vi "Realtime module.vi"() -> ()   [LabVIEW 2019]
uses:
  <vilib>/Platform/TimedLoop/XDataNode/timing_clust.ctl
  <vilib>/Platform/TimedLoop/XDataNode/nitl_modes.ctl
  <vilib>/Platform/TimedLoop/XDataNode/wakeup.ctl
  <vilib>/FPGAPlugInAG/myRIO-1900/niLvFpga_Open_myRIO-1900.vi
  <vilib>/rvi/interface/common/dynamic/niFpgaDynamicAddResources.vi
  <vilib>/Utility/error.llb/Error Cluster From Error Code.vi
  <vilib>/rvi/errors/niLvFpgaAdjustHostInterfaceError.vi
  <vilib>/FPGAPlugInAG/Dynamic/niLvFpga_Close_Dynamic.vi
  <vilib>/platform/TimedLoop/XDataNode/XDataNode.xnode
  <vilib>/rvi/interface/nirviOpenFPGA/nirviOpenFPGA.xnode
  FPGA Bitfiles/dcmotordynamomet_FPGATarget_FPGAmodule_FvbKT0KolIY.lvbitx
  FPGA module.vi
  <vilib>/rvi/interface/nirviMethod/nirviMethod.xnode
  <vilib>/rvi/interface/nirviCloseFPGA/nirviCloseFPGA.xnode
  <vilib>/FPGAPlugInAG/Dynamic/niLvFpga_ReadFifo_Dynamic.vi
  <vilib>/rvi/errors/niLvFpgaMergeErrorWithErrorCode.vi
  <vilib>/Platform/TimedLoop/XDataNode/XDNodeRunTimeDep.lvlib
  <vilib>/FPGAPlugInAG/Dynamic/niLvFpga_WriteFifo_Dynamic.vi
panel:
  in  "Ratio":sgl=0.4
  in  "Boolean":bool
  out "Error Chart":dynamicdata(graph)
  in  "Tab Control":T1(tab)
  out "?":dbl
  out "Slip":dbl(graph)
  out "?":dbl
  out "?":dbl
  out "AVG Speed (RPM)":dbl format="%#_5g"
  out "AVG Voltage Motor (V)":dbl format="%#_2g"
  out "AVG Voltage Battery (V)":dbl format="%#_4g"
  out "AVG Current Battery-Driver \nof Generator (A)":dbl format="%#_3g"
  out "AVG Current \nDriver-Generator (A)":dbl format="%#_2g"
  out "AVG Current Battery-Driver \nof Motor (A)":dbl format="%#_3g"
  out "AVG Current\nDriver-Motor (A)":dbl format="%#_3g"
  out "Lowpass Motor Voltage":dbl
  out "Current\nDriver-Generator (A)":dbl
  out "Current Battery-Driver\nof Generator (A)":dbl
  out "Current Battery-Driver\nof Motor (A)":dbl
  out "Current\nDriver-Motor (A)":dbl
  out "Generator Current Chart":dynamicdata(graph)
  in  "Generator\nCurrent (A)":dbl(slide) scale=0.0..40.0
  in  "Calibrated \nmax current":dbl=40.0
  in  "Motor\nVoltage (V)":dbl(slide) scale=0.0..24.0
  in  "Calibrated \nmax voltage":dbl=24.0
  out "Lowpass Battery Voltage":dbl
  out "Speed Chart":dynamicdata(graph)
  out "Voltage Chart":dynamicdata(graph)
  out "Motor Current Chart":dynamicdata(graph)
  out "AVG Motor Moment (Nm)":dbl format="%#_4g"
  out "AVG Generator Moment (Nm)":dbl format="%#_4g"
  out "Motor PID Chart":dynamicdata(graph)
  out "Generator PID Chart":dynamicdata(graph)
  out "b'":dbl
  out "a'":dbl
  out "b":dbl
  out "a":dbl
  in  "ELL":dbl=-0.8
  in  "EUL":dbl=0.8
  in  "EL1":dbl
  out "Error IN (G)":dbl
  out "Error OUT (G)":dbl
  out "Error In (M)":dbl
  out "Error OUT (M)":dbl
  in  "Alpha\nVoltage":dbl=0.05
  in  "Alpha\nCurrent":dbl=0.025
  in  "PID upper\n limit (G)":dbl
  in  "PID lower\n limit (G)":dbl=-1.0
  out "Output (G)":dbl
  out "PID (G)":dbl
  in  "I lower\nlimit (G)":dbl=-1.0
  in  "I upper\nlimit (G)":dbl
  out "D (G)":dbl
  out "I (G)":dbl
  out "P (G)":dbl
  in  "Kd (G)":dbl=0.001
  in  "Ki (G)":dbl=7.0
  in  "Kp (G)":dbl
  out "Output (M)":dbl
  in  "Kp (M)":dbl
  in  "Ki (M)":dbl=15.0
  in  "Kd (M)":dbl=0.01
  in  "I upper\nlimit (M)":dbl=1.0
  in  "I lower\nlimit (M)":dbl
  in  "PID lower\n limit (M)":dbl
  in  "PID upper\n limit (M)":dbl=1.0
  in  "PID Motor":bool=TRUE
  out "PID (M)":dbl
  in  "PID_Period\nMotor":dbl=0.005
  out "P (M)":dbl
  out "I (M)":dbl
  out "D (M)":dbl
  in  "PID Generator":bool=TRUE
  in  "PID_Period\nGenerator":dbl=0.005
  in  "Offset D-M":dbl
  in  "Offset B-D M":dbl
  in  "Offset D-G":dbl
  in  "Offset B-D G":dbl
  out "Output (Mot)":dbl
  out "C/Analog1":dbl
  out "C/Analog0":dbl
  out "A/Analog 3":dbl
  out "A/Analog2":dbl
  out "A/Analog1":dbl
  out "A/Analog0":dbl
  in  "C":dbl=5.1047
  in  "Min Channel C":dbl=-10.0
  in  "Min Channel A":dbl
  out "n samples":dbl
  out "Data 3":i32[](array[numeric]) caption="Data C/AI"
  in  "Max Channel C":dbl=10.0
  in  "B":dbl=-59.193
  in  "A":dbl=23.7
  in  "Max Channel A":dbl=5.0
  in  "Signal resolution":dbl=4095.0
  out "32bit integer generator":i32
  out "32bit integer motor":i32
  out "Samples":dbl
  out "Sum Bat Voltage":dbl
  out "Sum Mot Voltage":dbl
  out "Sum Bat-Dri of Gen":dbl
  out "Sum Bat-Dri of Mot":dbl
  out "Sum Generator":dbl
  out "Sum Motor":dbl
  out "Sum Speed":dbl
  in  "Encoder Resolution":dbl=16.0
  out "A/AI2":dbl
  out "A/AI3":dbl
  out "Executing Duration":u32
  out "Data":i32[](array[numeric])
  out "A/AI0":dbl
  out "A/AI1":dbl
  out "C/AI0":dbl
  out "Motor Voltage":dbl
  out "Bat-Dri Current (A) Mot":dbl
  out "Dri-Mot Current (A)":dbl
  out "Bat-Dri Current (A) Gen":dbl
  out "Dri-Gen Current (A)":dbl
  out "C/AI1":dbl
  out "Battery Voltage":dbl
  out "n speed":i32
  out "duration":i32
  out "Data Speed":i32[](array[numeric])
  out "Output (Gen)":dbl
  in  "Offset Motor Moment":dbl
  in  "Offset Generator Moment":dbl
  out "Motor Moment (Nm)":dbl format="%#_4g"
  out "Max Motor Moment":dbl
  out "Min Motor Moment":dbl
  out "Generator Moment (Nm)":dbl format="%#_4g"
  out "Max Gen Moment":dbl
  out "Min Gen Moment":dbl
  in  "alpha Motor moment":dbl=0.025
  in  "Lowpass Filter for Moment?":bool=TRUE
  in  "alpha Gen moment":dbl=0.025
  out "B/AI0":dbl
  out "B/AI1":dbl
  in  "Gain_Mot_Loadcell":dbl=3.6711
  in  "Offset_Mot_Loadcell":dbl=-8.6555
  in  "Gain_Gen_Loadcell":dbl=3.83101
  in  "Offset_Gen_Loadcell":dbl=-9.60463
  out "Sum ADC Mot Loadcell":dbl
  out "Sum ADC Gen Loadcell":dbl
  out "Sum Mot Moment":dbl
  out "Sum Gen Moment":dbl
  out "AVG ADC Mot Loadcell (V)":dbl
  out "AVG ADC Gen Loadcell (V)":dbl
  out "ADC B/AI0":dbl
  out "ADC B/AI1":dbl
  out "Motor Moment Chart":dbl(graph)
  out "Generator Moment Chart":dbl(graph)
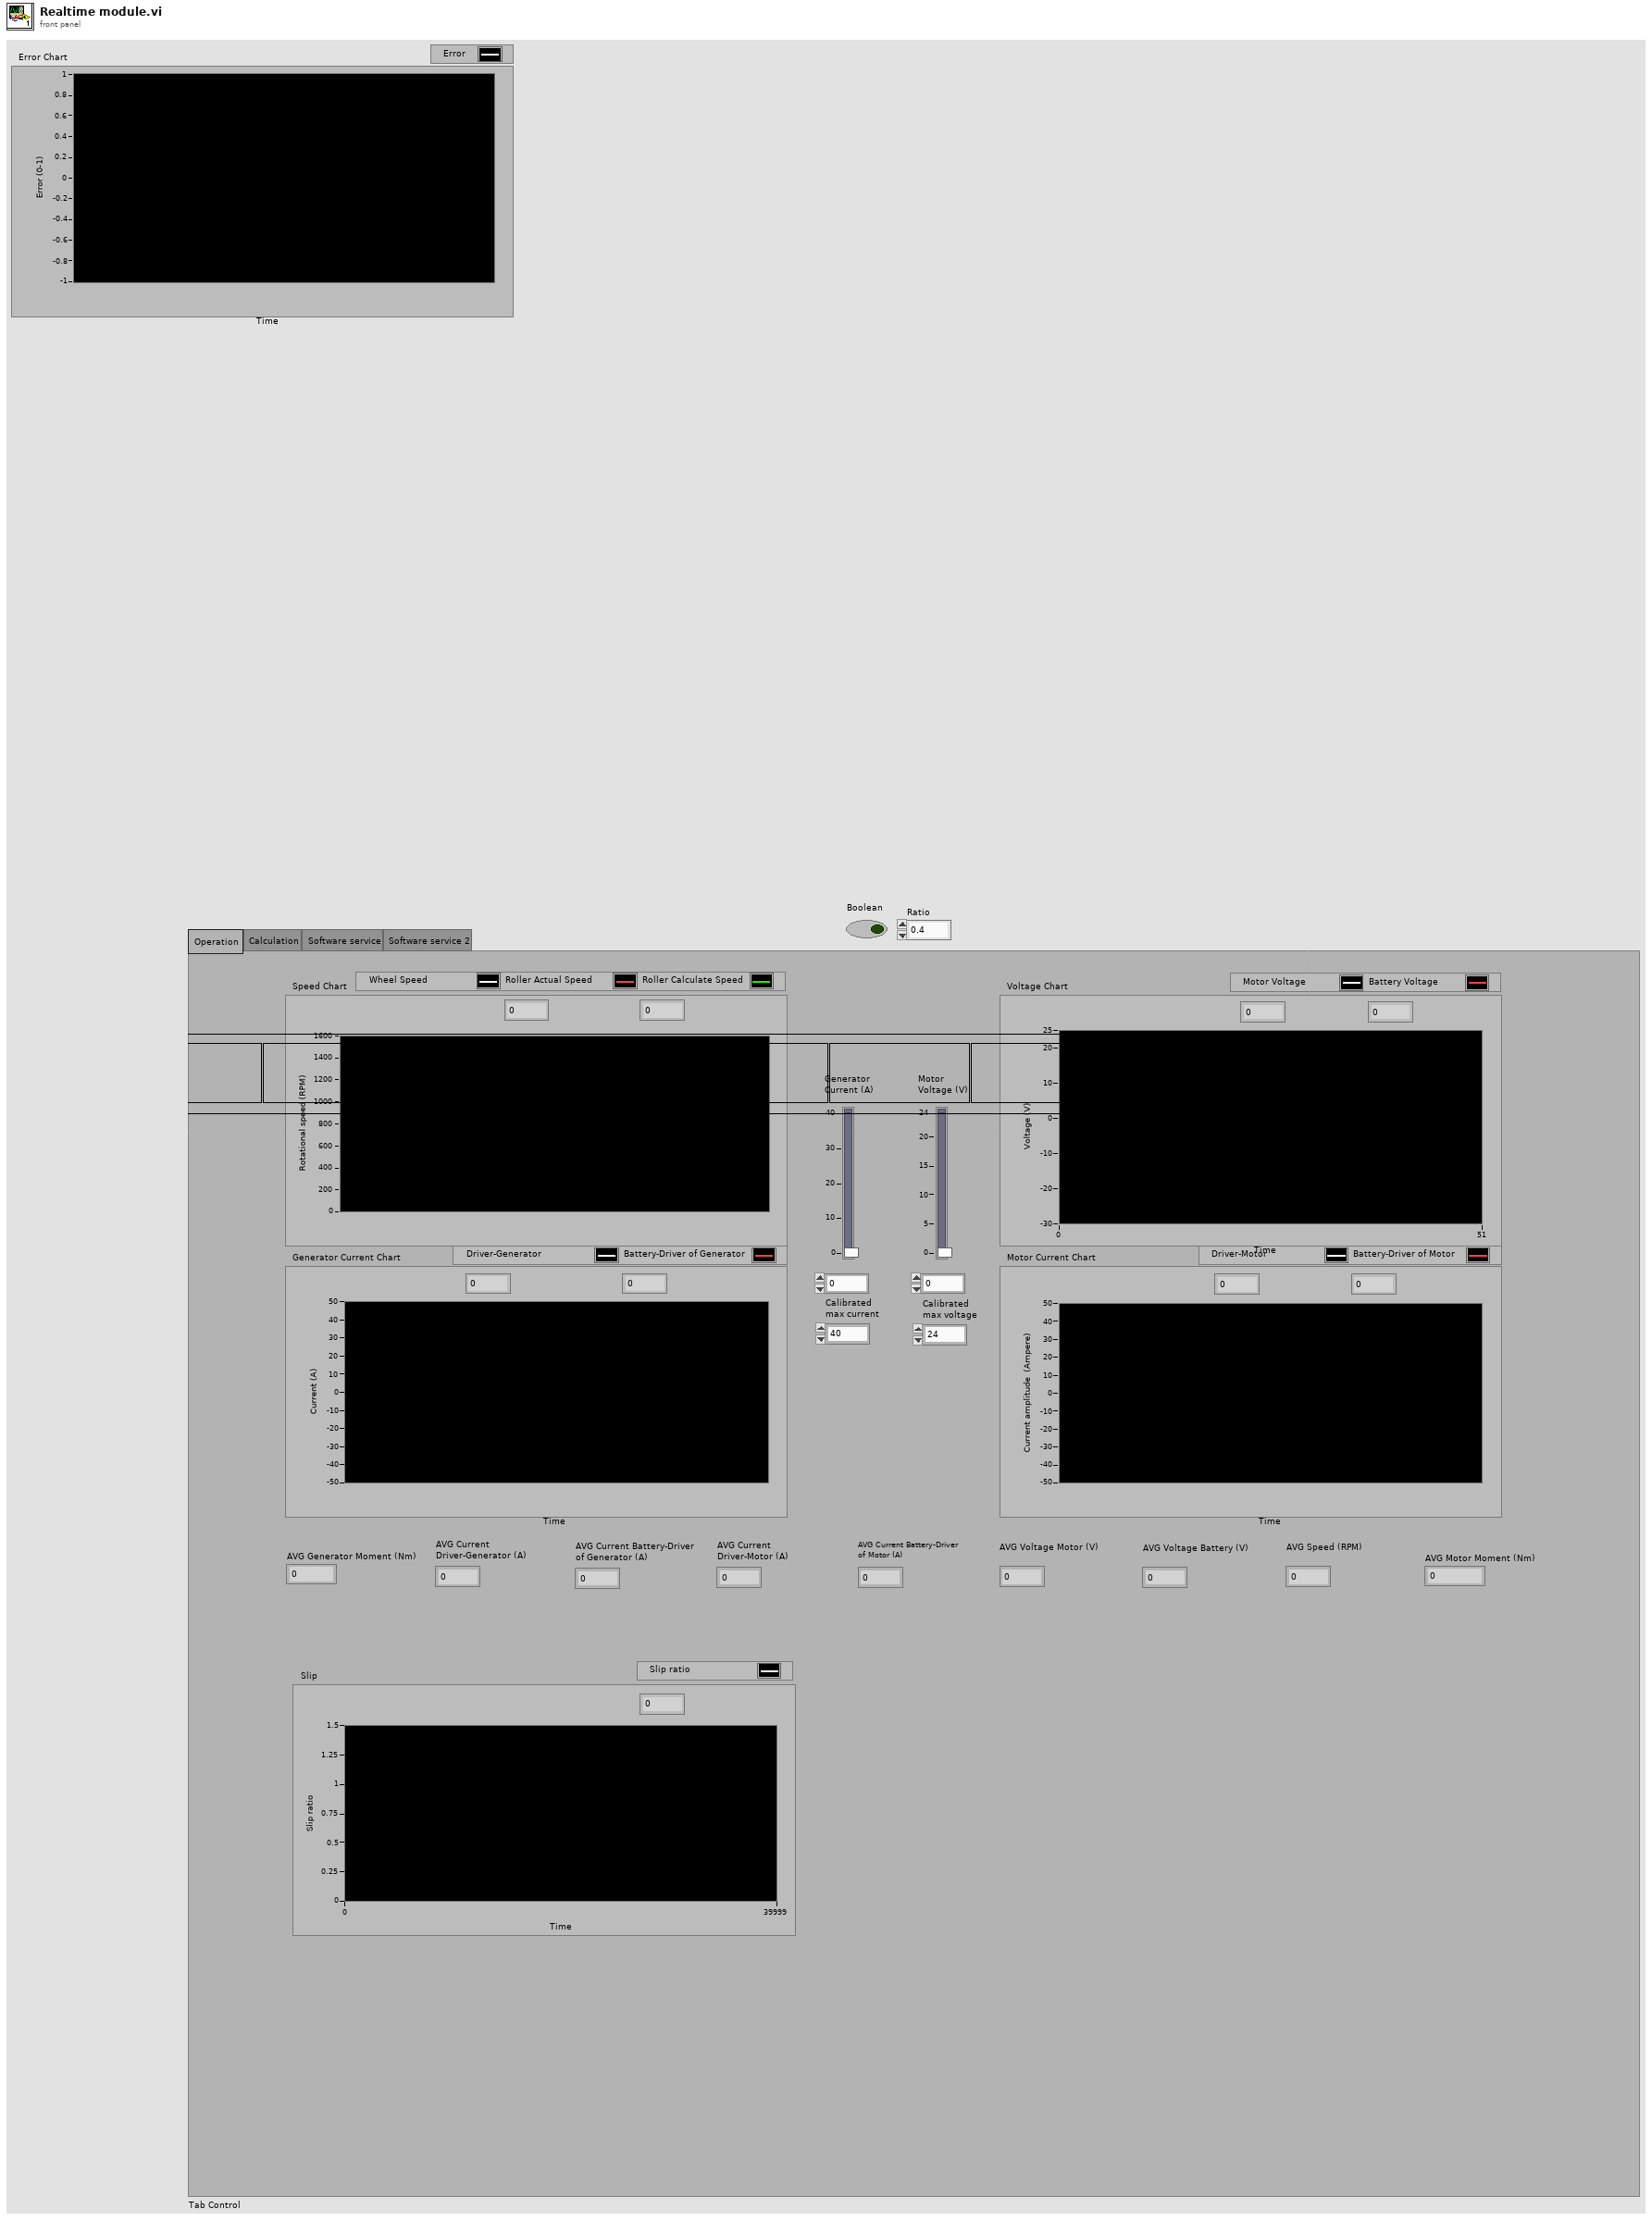
[diagram p1: front panel]
types:
  T1 = enum32{"Operation ", "Calculation", "Software service", "Software service 2"}
  T2 = typedef "XDNodeRunTimeDep.lvlib/timing_clust.ctl" = cluster{"Expected End [f-1]":u64, "Actual End [f-1]":u64, "Finished Late? [f-1]":bool, "Expected End [i-1]":u64, "Actual End [i-1]":u64, "Finished Late? [i-1]":bool, "Expected Start [i]":u64, "Actual Start [i]":u64, "Expected Start [f]":u64, "Actual Start [f]":u64, "Source Name":string, "Structure Name":string, "Period":i64, "Deadline":i64, "Offset":i64, "Start":i64, "Priority":i32, "Timeout":i32, "Mode":T3, "Wakeup Reason":T4, "Error":errorcluster, "Source Type":string, "Secondary Source Type":string, "Global End Time":u64, "Global Start Time":u64, "Frame Duration":u64, "Iteration Duration":u64, "Assigned CPU":i32, "I/O Scan Engine Mode":u32}
  T3 = typedef "XDNodeRunTimeDep.lvlib/nitl_modes.ctl" = enum32{"No Change", "Process missed periods, maintain original phase", "Discard missed periods, maintain original phase", "Process missed periods, ignore original phase", "Discard missed periods, ignore original phase"}
  T4 = typedef "XDNodeRunTimeDep.lvlib/wakeup.ctl" = enum32{"Normal", "Aborted", "Asynchronous wakeup", "Timing source error", "Timed loop error", "Timeout"}
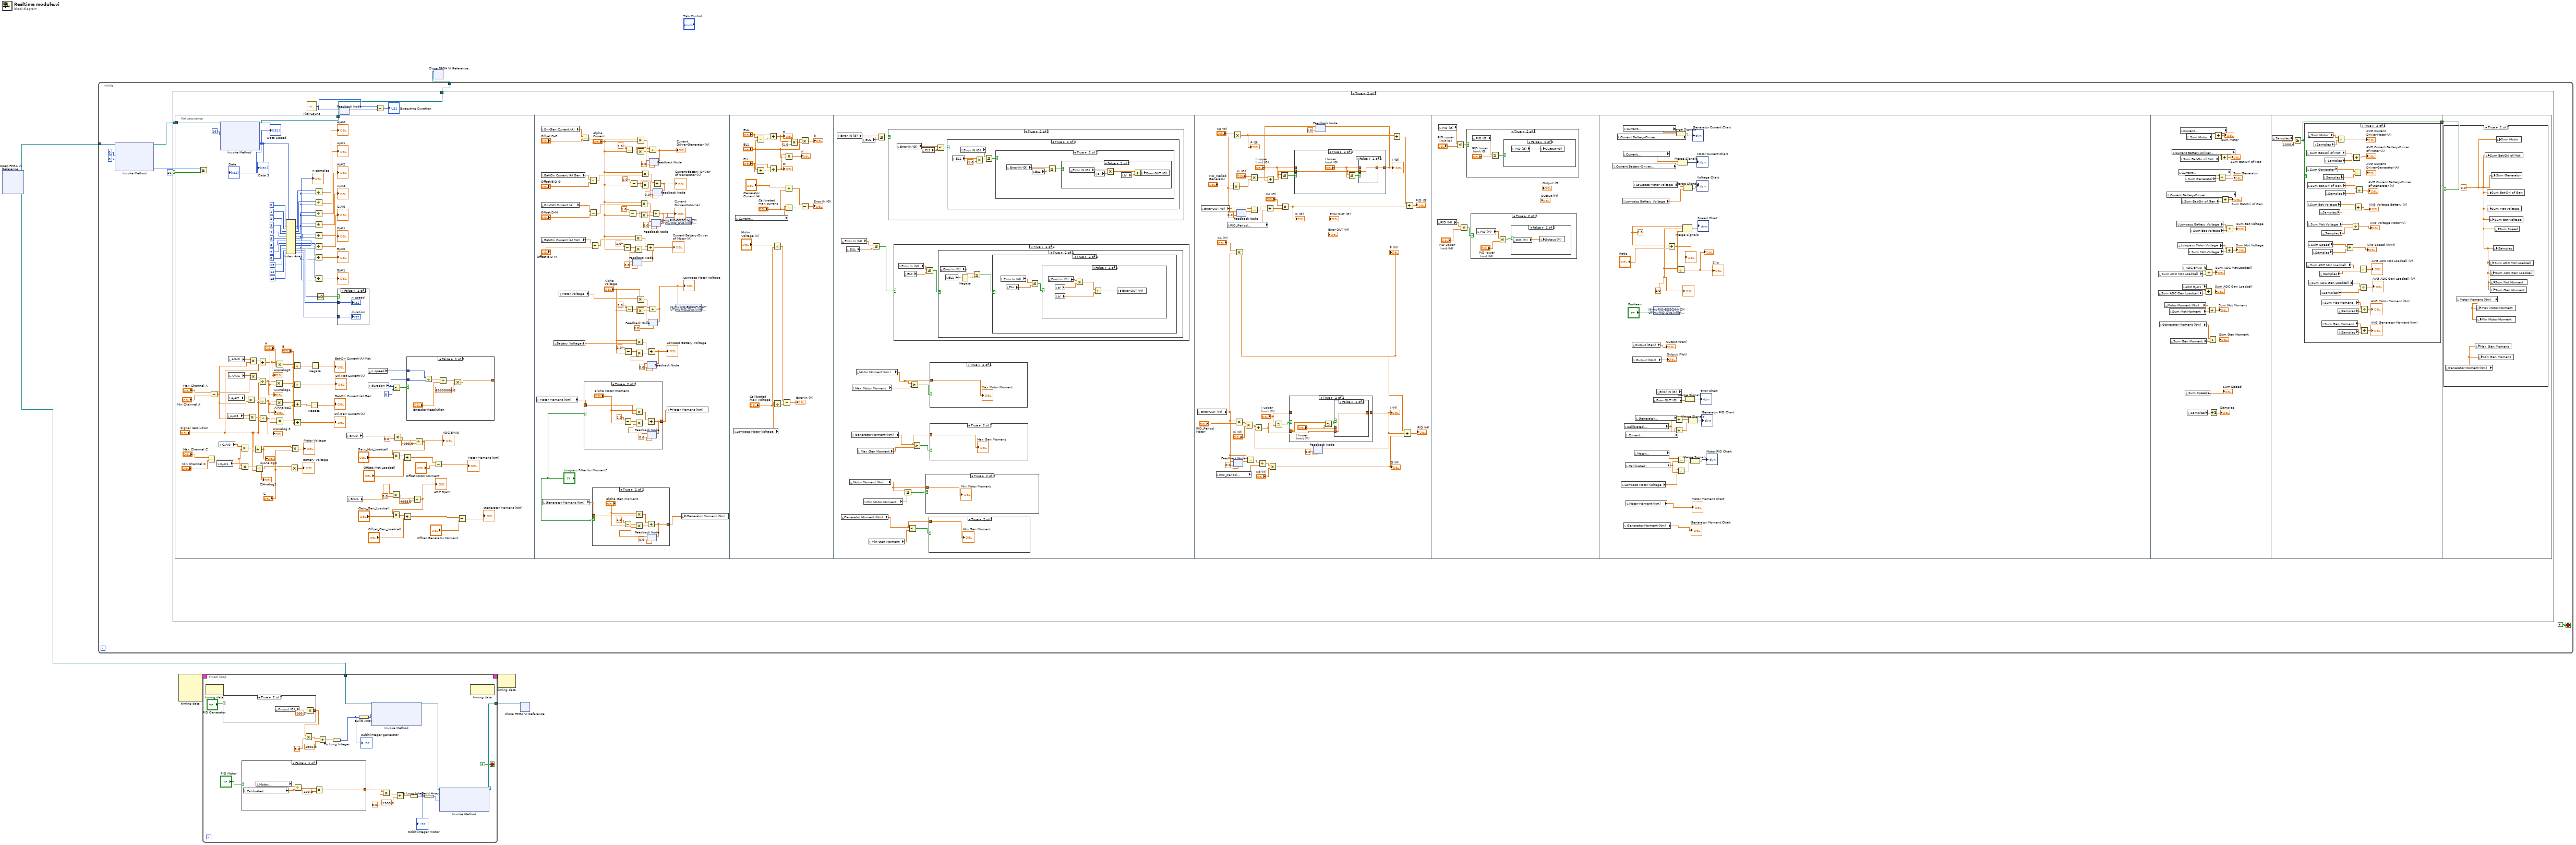
[diagram p0: block diagram]
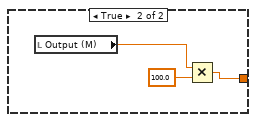
[diagram p2: hidden frame]
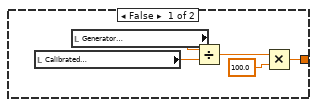
[diagram p3: hidden frame]
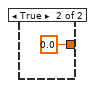
[diagram p5: hidden frame]
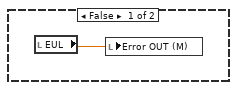
[diagram p13: hidden frame]
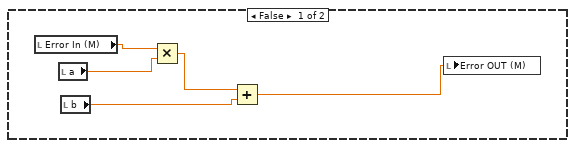
[diagram p14: hidden frame]
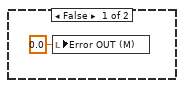
[diagram p15: hidden frame]
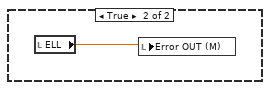
[diagram p16: hidden frame]
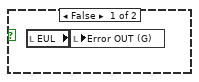
[diagram p17: hidden frame]
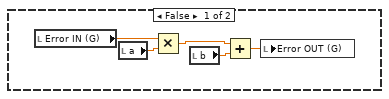
[diagram p18: hidden frame]
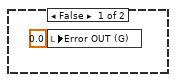
[diagram p19: hidden frame]
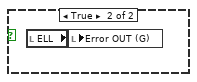
[diagram p20: hidden frame]
diagram:
  n1 = xnode "Open FPGA VI Reference"() -> ("FPGA VI Reference Out"=w1:refnum<k20>)  [unwired: 2 in, 1 out]
  n2 = while {
    tunnel: w1 -> [w14]
    tunnel: [w6] -> w2
    stop <- FALSE stop-if-true
    n3 = xnode "Invoke Method"("FPGA VI Reference In"=w14, "Number of Elements"=u32 0, "Timeout (ms)"=0) -> ("FPGA VI Reference Out"=w11:refnum<k20>, "Elements Remaining"=w7:u32)  [unwired: 1 in, 2 out]
    n4 = Greater Or Equal?(x=w7, y=u32 16) -> (x >= y?=w12:bool)
    n5 = case shown="True" w12 {
      tunnel: w11 -> [w15 w21]
      tunnel: [w15 w17] -> w6
      frame False {
      }
      frame True {
        n6 = flat-sequence {
          tunnel: w21 -> [w124]
          tunnel: [w115] -> w17
          tunnel: [w453] -> w16
          tunnel: w16 -> [w489]
          frame #0 {
            n7 = Subtract(x="Max Channel C", y="Min Channel C") -> (x-y=w80:dbl)
            n8 = Subtract(x="Max Channel A", y="Min Channel A") -> (x-y=w71:dbl)
            n9 = local read "C/AI1"() -> (w81:dbl)
            n10 = local read "C/AI0"() -> (w82:dbl)
            n11 = xnode "Invoke Method"("FPGA VI Reference In"=w124, "Number of Elements"=u32 16) -> ("FPGA VI Reference Out"=w115:refnum<k20>, "Data"=w85:i32[])  [unwired: 2 in, 2 out]
            "Data" <- w85
            "Data Speed" <- w85
            "Data 3" <- w85
            n12 = local read "A/AI3"() -> (w72:dbl)
            n13 = local read "A/AI2"() -> (w73:dbl)
            n14 = local read "A/AI0"() -> (w75:dbl)
            n15 = local read "A/AI1"() -> (w74:dbl)
            n16 = Multiply(x=w82, y=w80) -> (x*y=w79:dbl)
            n17 = Multiply(x=w81, y=w80) -> (x*y=w78:dbl)
            n18 = Multiply(x=w73, y=w71) -> (x*y=w68:dbl)
            n19 = Multiply(x=w72, y=w71) -> (x*y=w67:dbl)
            n20 = Multiply(x=w75, y=w71) -> (x*y=w70:dbl)
            n21 = Multiply(x=w74, y=w71) -> (x*y=w69:dbl)
            n22 = Divide(x=w79, y="Signal resolution") -> (x/y=w57:dbl)
            "C/Analog0" <- w57
            n23 = Divide(x=w78, y="Signal resolution") -> (x/y=w58:dbl)
            "C/Analog1" <- w58
            n24 = Divide(x=w70, y="Signal resolution") -> (x/y=w59:dbl)
            "A/Analog0" <- w59
            n25 = Divide(x=w69, y="Signal resolution") -> (x/y=w60:dbl)
            "A/Analog1" <- w60
            n26 = Divide(x=w68, y="Signal resolution") -> (x/y=w61:dbl)
            "A/Analog2" <- w61
            n27 = Divide(x=w67, y="Signal resolution") -> (x/y=w62:dbl)
            "A/Analog 3" <- w62
            n28 = Multiply(x=w60, y="A") -> (x*y=w105:dbl)
            n29 = Multiply(x=w61, y="A") -> (x*y=w117:dbl)
            n30 = Multiply(x=w59, y="A") -> (x*y=w106:dbl)
            n31 = Multiply(x=w62, y="A") -> (x*y=w116:dbl)
            n32 = Index Array(array=w85, index #1=0 ("index"), index #2=1 ("index"), index #3=2 ("index"), index #4=3 ("index"), index #5=4 ("index"), index #6=5 ("index"), index #7=6 ("index"), index #8=7 ("index"), index #9=8 ("index"), index #10=13 ("index"), index #11=14 ("index"), index #12=15 ("index")) -> (element #1=w38:i32, element #2=w110:i32, element #3=w109:i32, element #4=w108:i32, element #5=w107:i32, element #6=w100:i32, element #7=w91:i32, element #8=w40:i32, element #9=w39:i32, element #10=w51:i32, element #11=w52:i32, element #12=w53:i32)
            "n samples" <- w38
            n33 = Multiply(x=w58, y="C") -> (x*y=→"Battery Voltage":dbl)
            n34 = Multiply(x=w57, y="C") -> (x*y=→"Motor Voltage":dbl)
            n35 = Add(x=w106, y="B") -> (x+y=w104:dbl)
            n36 = Add(x=w105, y="B") -> (x+y=→"Dri-Mot Current (A)":dbl)
            n37 = Add(x=w117, y="B") -> (x+y=w89:dbl)
            n38 = Add(x=w116, y="B") -> (x+y=→"Dri-Gen Current (A)":dbl)
            n39 = Negate(x=w89) -> (-x=→"Bat-Dri Current (A) Gen":dbl)
            n40 = Negate(x=w104) -> (-x=→"Bat-Dri Current (A) Mot":dbl)
            n41 = Divide(x=w110, y=w38) -> (x/y=→"A/AI0":dbl)
            n42 = Divide(x=w109, y=w38) -> (x/y=→"A/AI1":dbl)
            n43 = Divide(x=w108, y=w38) -> (x/y=→"A/AI2":dbl)
            n44 = Divide(x=w107, y=w38) -> (x/y=→"A/AI3":dbl)
            n45 = Divide(x=w100, y=w38) -> (x/y=→"C/AI0":dbl)
            n46 = Divide(x=w91, y=w38) -> (x/y=→"C/AI1":dbl)
            n47 = Divide(x=w40, y=w38) -> (x/y=→"B/AI0":dbl)
            n48 = Divide(x=w39, y=w38) -> (x/y=→"B/AI1":dbl)
            n49 = Equal To 0?(x=w51) -> (x = 0?=w97:bool)
            n50 = case shown="False" w97 {
              tunnel: w52 -> [w134 _]
              tunnel: w53 -> [w133 _]
              frame False {
                "n speed" <- w134
                "duration" <- w133
              }
              frame True {
              }
            }
            n51 = local read "B/AI0"() -> (w37:dbl)
            n52 = local read "B/AI1"() -> (w29:dbl)
            n53 = local read "n speed"() -> (w95:i32)
            n54 = local read "duration"() -> (w94:i32)
            n55 = Multiply(x=w29, y=5.0) -> (x*y=w31:dbl)
            n56 = Less Or Equal?(x=w94, y=0) -> (x <= y?=w93:bool)
            n57 = Multiply(x=w37, y=5.0) -> (x*y=w35:dbl)
            n58 = case shown="False" w93 {
              tunnel: w95 -> [w128 _]
              tunnel: w94 -> [w127 _]
              tunnel: [w125 0.0] -> _
              frame False {
                n59 = Divide(x=w128, y=w127) -> (x/y=w130:dbl)
                n60 = Divide(x=w130, y="Encoder Resolution") -> (x/y=w131:dbl)
                n61 = Multiply(x=w131, y=60000000.0) -> (x*y=w125:dbl)
              }
              frame True {
              }
            }
            n62 = Divide(x=w31, y=4095.0) -> (x/y=w28:dbl)
            "ADC B/AI1" <- w28
            n63 = Multiply(x=w28, y="Gain_Gen_Loadcell") -> (x*y=w43:dbl)
            n64 = Add(x=w43, y="Offset_Gen_Loadcell") -> (x+y=w24:dbl)
            n65 = Divide(x=w35, y=4095.0) -> (x/y=w33:dbl)
            "ADC B/AI0" <- w33
            n66 = Multiply(x=w33, y="Gain_Mot_Loadcell") -> (x*y=w46:dbl)
            n67 = Add(x=w46, y="Offset_Mot_Loadcell") -> (x+y=w27:dbl)
            n68 = Subtract(x=w27, y="Offset Motor Moment") -> (x-y=→"Motor Moment (Nm)":dbl)
            n69 = Subtract(x=w24, y="Offset Generator Moment") -> (x-y=→"Generator Moment (Nm)":dbl)
          }
          frame #1 {
            n70 = local read "Motor Moment (Nm)"() -> (w150:dbl)
            n71 = local read "Dri-Gen Current (A)"() -> (w136:dbl)
            n72 = local read "Bat-Dri Current (A) Gen"() -> (w139:dbl)
            n73 = local read "Dri-Mot Current (A)"() -> (w142:dbl)
            n74 = local read "Bat-Dri Current (A) Mot"() -> (w145:dbl)
            n75 = local read "Generator Moment (Nm)"() -> (w149:dbl)
            n76 = local read "Battery Voltage"() -> (w153:dbl)
            n77 = local read "Motor Voltage"() -> (w161:dbl)
            n78 = Subtract(x=w136, y="Offset D-G") -> (x-y=w137:dbl)
            n79 = case shown="True" "Lowpass Filter for Moment?" {
              tunnel: [w208 w210] -> w151
              tunnel: w150 -> [w208 w209]
              frame False {
              }
              frame True {
                n80 = Subtract(x=1.0, y="alpha Motor moment") -> (x-y=w216:dbl)
                n81 = Multiply(x="alpha Motor moment", y=w209) -> (x*y=w217:dbl)
                n82 = feedback #1(0.0) -> (w214:dbl)
                n83 = Multiply(x=w216, y=w214) -> (x*y=w213:dbl)
                n84 = Add(x=w217, y=w213) -> (x+y=w210:dbl)
                n85 = feedback-in #1(w210) -> ()
              }
            }
            n86 = Subtract(x=w139, y="Offset B-D G") -> (x-y=w140:dbl)
            n87 = Subtract(x=w142, y="Offset D-M") -> (x-y=w143:dbl)
            n88 = Subtract(x=w145, y="Offset B-D M") -> (x-y=w146:dbl)
            n89 = case shown="True" "Lowpass Filter for Moment?" {
              tunnel: w149 -> [w198 w200]
              tunnel: [w198 w199] -> w148
              frame False {
              }
              frame True {
                n90 = Subtract(x=1.0, y="alpha Gen moment") -> (x-y=w206:dbl)
                n91 = Multiply(x="alpha Gen moment", y=w200) -> (x*y=w207:dbl)
                n92 = feedback #2(0.0) -> (w204:dbl)
                n93 = Multiply(x=w206, y=w204) -> (x*y=w203:dbl)
                n94 = Add(x=w207, y=w203) -> (x+y=w199:dbl)
                n95 = feedback-in #2(w199) -> ()
              }
            }
            n96 = Subtract(x=1.0, y="Alpha\nCurrent") -> (x-y=w178:dbl)
            n97 = Subtract(x=1.0, y="Alpha\nVoltage") -> (x-y=w159:dbl)
            n98 = Subtract(x=1.0, y="Alpha\nCurrent") -> (x-y=w196:dbl)
            n99 = Subtract(x=1.0, y="Alpha\nVoltage") -> (x-y=w167:dbl)
            n100 = Subtract(x=1.0, y="Alpha\nCurrent") -> (x-y=w184:dbl)
            n101 = Subtract(x=1.0, y="Alpha\nCurrent") -> (x-y=w190:dbl)
            n102 = feedback #3(0.0) -> (w175:dbl)
            n103 = Multiply(x="Alpha\nCurrent", y=w146) -> (x*y=w179:dbl)
            n104 = Multiply(x=w178, y=w175) -> (x*y=w174:dbl)
            n105 = Multiply(x="Alpha\nVoltage", y=w153) -> (x*y=w160:dbl)
            n106 = Multiply(x=w137, y="Alpha\nCurrent") -> (x*y=w197:dbl)
            n107 = Multiply(x=w161, y="Alpha\nVoltage") -> (x*y=w168:dbl)
            n108 = Multiply(x="Alpha\nCurrent", y=w143) -> (x*y=w185:dbl)
            n109 = Multiply(x="Alpha\nCurrent", y=w140) -> (x*y=w191:dbl)
            n110 = Add(x=w179, y=w174) -> (x+y=w176:dbl)
            "Current Battery-Driver\nof Motor (A)" <- w176
            n111 = feedback-in #3(w176) -> ()
            n112 = feedback #4(0.0) -> (w156:dbl)
            n113 = Multiply(x=w159, y=w156) -> (x*y=w155:dbl)
            n114 = Add(x=w160, y=w155) -> (x+y=w157:dbl)
            "Lowpass Battery Voltage" <- w157
            n115 = feedback-in #4(w157) -> ()
            n116 = feedback #5(0.0) -> (w164:dbl)
            n117 = Multiply(x=w167, y=w164) -> (x*y=w163:dbl)
            n118 = Add(x=w168, y=w163) -> (x+y=w165:dbl)
            "Lowpass Motor Voltage" <- w165
            n119 = feedback-in #5(w165) -> ()
            n120 = feedback #6(0.0) -> (w193:dbl)
            n121 = Multiply(x=w196, y=w193) -> (x*y=w192:dbl)
            n122 = Add(x=w197, y=w192) -> (x+y=w194:dbl)
            "Current\nDriver-Generator (A)" <- w194
            n123 = feedback-in #6(w194) -> ()
            n124 = feedback #7(0.0) -> (w181:dbl)
            n125 = Multiply(x=w184, y=w181) -> (x*y=w180:dbl)
            n126 = Add(x=w185, y=w180) -> (x+y=w182:dbl)
            "Current\nDriver-Motor (A)" <- w182
            n127 = feedback-in #7(w182) -> ()
            n128 = feedback #8(0.0) -> (w187:dbl)
            n129 = Multiply(x=w190, y=w187) -> (x*y=w186:dbl)
            n130 = Add(x=w191, y=w186) -> (x+y=w188:dbl)
            "Current Battery-Driver\nof Generator (A)" <- w188
            n131 = feedback-in #8(w188) -> ()
            n132 = shared-variable "NI-myRIO-BOSCH-HCMUT\\myRIO_SVs.lvlib\\Current"(w182) -> ()  [unwired: 1 in, 1 out]
            n133 = local write "Motor Moment (Nm)"(w151) -> ()
            n134 = shared-variable "NI-myRIO-BOSCH-HCMUT\\myRIO_SVs.lvlib\\Voltage"(w165) -> ()  [unwired: 1 in, 1 out]
            n135 = local write "Generator Moment (Nm)"(w148) -> ()
          }
          frame #2 {
            n136 = local read "Lowpass Motor Voltage"() -> (w222:dbl)
            n137 = local read "Current\nDriver-Generator (A)"() -> (w218:dbl)
            n138 = Subtract(x="EUL", y="EL1") -> (x-y=w237:dbl)
            n139 = Add(x="EL1", y="ELL") -> (x+y=w231:dbl)
            n140 = Divide(x="EUL", y=w237) -> (x/y=w233:dbl)
            "a" <- w233
            n141 = Divide(x="ELL", y=w231) -> (x/y=w229:dbl)
            "a'" <- w229
            n142 = Divide(x="Motor\nVoltage (V)", y="Calibrated \nmax voltage") -> (x/y=w221:dbl)
            n143 = Divide(x=w222, y="Calibrated \nmax voltage") -> (x/y=w220:dbl)
            n144 = Subtract(x=w221, y=w220) -> (x-y=→"Error In (M)":dbl)
            n145 = Multiply(x=w229, y="EL1") -> (x*y=→"b'":dbl)
            n146 = Divide(x="Generator\nCurrent (A)", y="Calibrated \nmax current") -> (x/y=w240:dbl)
            n147 = Divide(x=w218, y="Calibrated \nmax current") -> (x/y=w239:dbl)
            n148 = Multiply(x=w233, y=-1.0) -> (x*y=w234:dbl)
            n149 = Multiply(x="EL1", y=w234) -> (x*y=→"b":dbl)
            n150 = Subtract(x=w240, y=w239) -> (x-y=→"Error IN (G)":dbl)
          }
          frame #3 {
            n151 = local read "Error IN (G)"() -> (w258:dbl)
            n152 = local read "Generator Moment (Nm)"() -> (w241:dbl)
            n153 = local read "Error In (M)"() -> (w255:dbl)
            n154 = local read "EUL"() -> (w254:dbl)
            n155 = local read "Motor Moment (Nm)"() -> (w243:dbl)
            n156 = local read "Generator Moment (Nm)"() -> (w247:dbl)
            n157 = local read "Max Motor Moment"() -> (w252:dbl)
            n158 = local read "Motor Moment (Nm)"() -> (w250:dbl)
            n159 = local read "Max Gen Moment"() -> (w249:dbl)
            n160 = local read "EUL"() -> (w257:dbl)
            n161 = local read "Min Motor Moment"() -> (w246:dbl)
            n162 = local read "Min Gen Moment"() -> (w245:dbl)
            n163 = Less Or Equal?(x=w255, y=w254) -> (x <= y?=w253:bool)
            n164 = Less Or Equal?(x=w258, y=w257) -> (x <= y?=w256:bool)
            n165 = case shown="True" w256 {
              frame False {
                n166 = local read "EUL"() -> (w286:dbl)
                n167 = local write "Error OUT (G)"(w286) -> ()
              }
              frame True {
                n168 = local read "Error IN (G)"() -> (w289:dbl)
                n169 = local read "EL1"() -> (w288:dbl)
                n170 = Less Or Equal?(x=w289, y=w288) -> (x <= y?=w287:bool)
                n171 = case shown="True" w287 {
                  frame False {
                    n172 = local read "Error IN (G)"() -> (w294:dbl)
                    n173 = local read "a"() -> (w293:dbl)
                    n174 = Multiply(x=w294, y=w293) -> (x*y=w292:dbl)
                    n175 = local read "b"() -> (w291:dbl)
                    n176 = Add(x=w292, y=w291) -> (x+y=w290:dbl)
                    n177 = local write "Error OUT (G)"(w290) -> ()
                  }
                  frame True {
                    n178 = local read "EL1"() -> (w299:dbl)
                    n179 = local read "Error IN (G)"() -> (w296:dbl)
                    n180 = Multiply(x=w299, y=-1.0) -> (x*y=w297:dbl)
                    n181 = Less Or Equal?(x=w296, y=w297) -> (x <= y?=w295:bool)
                    n182 = case shown="True" w295 {
                      frame False {
                        n183 = local write "Error OUT (G)"(0.0 ("Error OUT")) -> ()
                      }
                      frame True {
                        n184 = local read "Error IN (G)"() -> (w303:dbl)
                        n185 = local read "ELL"() -> (w302:dbl)
                        n186 = Less Or Equal?(x=w303, y=w302) -> (x <= y?=w301:bool)
                        n187 = case shown="False" w301 {
                          frame False {
                            n188 = local read "Error IN (G)"() -> (w308:dbl)
                            n189 = local read "a'"() -> (w307:dbl)
                            n190 = Multiply(x=w308, y=w307) -> (x*y=w306:dbl)
                            n191 = local read "b'"() -> (w305:dbl)
                            n192 = Add(x=w306, y=w305) -> (x+y=w304:dbl)
                            n193 = local write "Error OUT (G)"(w304) -> ()
                          }
                          frame True {
                            n194 = local read "ELL"() -> (w309:dbl)
                            n195 = local write "Error OUT (G)"(w309) -> ()
                          }
                        }
                      }
                    }
                  }
                }
              }
            }
            n196 = case shown="True" w253 {
              frame False {
                n197 = local read "EUL"() -> (w263:dbl)
                n198 = local write "Error OUT (M)"(w263) -> ()
              }
              frame True {
                n199 = local read "Error In (M)"() -> (w266:dbl)
                n200 = local read "EL1"() -> (w265:dbl)
                n201 = Less Or Equal?(x=w266, y=w265) -> (x <= y?=w264:bool)
                n202 = case shown="True" w264 {
                  frame False {
                    n203 = local read "Error In (M)"() -> (w271:dbl)
                    n204 = local read "a"() -> (w270:dbl)
                    n205 = local read "b"() -> (w268:dbl)
                    n206 = Multiply(x=w271, y=w270) -> (x*y=w269:dbl)
                    n207 = Add(x=w269, y=w268) -> (x+y=w267:dbl)
                    n208 = local write "Error OUT (M)"(w267) -> ()
                  }
                  frame True {
                    n209 = local read "Error In (M)"() -> (w274:dbl)
                    n210 = local read "EL1"() -> (w275:dbl)
                    n211 = Negate(x=w275) -> (-x=w273:dbl)
                    n212 = Less Or Equal?(x=w274, y=w273) -> (x <= y?=w272:bool)
                    n213 = case shown="True" w272 {
                      frame False {
                        n214 = local write "Error OUT (M)"(0.0 ("Error OUT (V)")) -> ()
                      }
                      frame True {
                        n215 = local read "Error In (M)"() -> (w279:dbl)
                        n216 = local read "ELL"() -> (w278:dbl)
                        n217 = Less Or Equal?(x=w279, y=w278) -> (x <= y?=w277:bool)
                        n218 = case shown="False" w277 {
                          frame False {
                            n219 = local read "Error In (M)"() -> (w284:dbl)
                            n220 = local read "a'"() -> (w283:dbl)
                            n221 = local read "b'"() -> (w282:dbl)
                            n222 = Multiply(x=w284, y=w283) -> (x*y=w281:dbl)
                            n223 = Add(x=w281, y=w282) -> (x+y=w280:dbl)
                            n224 = local write "Error OUT (M)"(w280) -> ()
                          }
                          frame True {
                            n225 = local read "ELL"() -> (w285:dbl)
                            n226 = local write "Error OUT (M)"(w285) -> ()
                          }
                        }
                      }
                    }
                  }
                }
              }
            }
            n227 = Less Or Equal?(x=w243, y=w246) -> (x <= y?=w244:bool)
            n228 = Less Or Equal?(x=w241, y=w245) -> (x <= y?=w242:bool)
            n229 = Greater Or Equal?(x=w250, y=w252) -> (x >= y?=w251:bool)
            n230 = Greater Or Equal?(x=w247, y=w249) -> (x >= y?=w248:bool)
            n231 = case shown="True" w244 {
              tunnel: w243 -> [_ w260]
              frame False {
              }
              frame True {
                "Min Motor Moment" <- w260
              }
            }
            n232 = case shown="True" w242 {
              tunnel: w241 -> [_ w259]
              frame False {
              }
              frame True {
                "Min Gen Moment" <- w259
              }
            }
            n233 = case shown="True" w248 {
              tunnel: w247 -> [_ w261]
              frame False {
              }
              frame True {
                "Max Gen Moment" <- w261
              }
            }
            n234 = case shown="True" w251 {
              tunnel: w250 -> [_ w262]
              frame False {
              }
              frame True {
                "Max Motor Moment" <- w262
              }
            }
          }
          frame #4 {
            n235 = local read "Error OUT (M)"() -> (w320:dbl)
            n236 = local read "Error OUT (G)"() -> (w339:dbl)
            n237 = local read "PID_Period\nMotor"() -> (w318:dbl)
            n238 = local read "PID_Period\nGenerator"() -> (w311:dbl)
            n239 = Multiply(x="PID_Period\nGenerator", y=w339) -> (x*y=w337:dbl)
            n240 = Multiply(x="Kp (G)", y=w339) -> (x*y=w346:dbl)
            "P (G)" <- w346
            n241 = feedback-in #9(w320) -> ()
            n242 = feedback #9(0.0 ("Error OUT (V)")) -> (w322:dbl)
            n243 = Multiply(x=w320, y="PID_Period\nMotor") -> (x*y=w330:dbl)
            n244 = Multiply(x="Kp (M)", y=w320) -> (x*y=w315:dbl)
            "P (M)" <- w315
            n245 = feedback-in #10(w339) -> ()
            n246 = feedback #10(0.0 ("Error OUT")) -> (w350:dbl)
            n247 = Multiply(x=w330, y="Ki (M)") -> (x*y=w328:dbl)
            n248 = Subtract(x=w320, y=w322) -> (x-y=w319:dbl)
            n249 = Multiply(x="Ki (G)", y=w337) -> (x*y=w335:dbl)
            n250 = Subtract(x=w339, y=w350) -> (x-y=w310:dbl)
            n251 = Divide(x=w319, y=w318) -> (x/y=w317:dbl)
            n252 = Divide(x=w310, y=w311) -> (x/y=w347:dbl)
            n253 = Multiply(x=w317, y="Kd (M)") -> (x*y=w313:dbl)
            "D (M)" <- w313
            n254 = Multiply(x="Kd (G)", y=w347) -> (x*y=w343:dbl)
            "D (G)" <- w343
            n255 = feedback #11(0.0 ("I upper limit (V)")) -> (w324:dbl)
            n256 = Add(x=w328, y=w324) -> (x+y=w326:dbl)
            n257 = Less Or Equal?(x=w326, y="I upper\nlimit (M)") -> (x <= y?=w327:bool)
            n258 = case shown="True" w327 {
              tunnel: w326 -> [_ w356]
              tunnel: "I upper\nlimit (M)" -> [w353 _]
              tunnel: [w353 w355] -> w314
              frame False {
              }
              frame True {
                n259 = Less Or Equal?(x=w356, y="I lower\nlimit (M)") -> (x <= y?=w357:bool)
                n260 = case shown="False" w357 {
                  tunnel: w356 -> [w358 _]
                  tunnel: [w358 w359] -> w355
                  tunnel: "I lower\nlimit (M)" -> [_ w359]
                  frame False {
                  }
                  frame True {
                  }
                }
              }
            }
            "I (M)" <- w314
            n261 = feedback-in #11(w314) -> ()
            n262 = feedback #12(0.0) -> (w334:dbl)
            n263 = Add(x=w335, y=w334) -> (x+y=w333:dbl)
            n264 = Less Or Equal?(x=w333, y="I upper\nlimit (G)") -> (x <= y?=w340:bool)
            n265 = case shown="True" w340 {
              tunnel: "I upper\nlimit (G)" -> [w360 _]
              tunnel: [w360 w362] -> w345
              tunnel: w333 -> [_ w361]
              frame False {
              }
              frame True {
                n266 = Less Or Equal?(x=w361, y="I lower\nlimit (G)") -> (x <= y?=w364:bool)
                n267 = case shown="False" w364 {
                  tunnel: [w365 w366] -> w362
                  tunnel: "I lower\nlimit (G)" -> [_ w366]
                  tunnel: w361 -> [w365 _]
                  frame False {
                  }
                  frame True {
                  }
                }
              }
            }
            "I (G)" <- w345
            n268 = feedback-in #12(w345) -> ()
            n269 = Add(x=w346, y=w345) -> (x+y=w344:dbl)
            n270 = Compound Arithmetic op=ADD(w315, w314, w313) -> (→"PID (M)":dbl)
            n271 = Add(x=w344, y=w343) -> (x+y=→"PID (G)":dbl)
          }
          frame #5 {
            n272 = local read "PID (M)"() -> (w369:dbl)
            n273 = local read "PID (G)"() -> (w371:dbl)
            n274 = Less Or Equal?(x=w371, y="PID upper\n limit (G)") -> (x <= y?=w370:bool)
            n275 = Less Or Equal?(x=w369, y="PID upper\n limit (M)") -> (x <= y?=w367:bool)
            n276 = case shown="True" w370 {
              frame False {
                n277 = local read "PID upper\n limit (G)"() -> (w379:dbl)
                n278 = local write "Output (G)"(w379) -> ()
              }
              frame True {
                n279 = local read "PID (G)"() -> (w382:dbl)
                n280 = Less Or Equal?(x=w382, y="PID lower\n limit (G)") -> (x <= y?=w380:bool)
                n281 = case shown="False" w380 {
                  frame False {
                    n282 = local read "PID (G)"() -> (w383:dbl)
                    n283 = local write "Output (G)"(w383) -> ()
                  }
                  frame True {
                    n284 = local read "PID lower\n limit (G)"() -> (w384:dbl)
                    n285 = local write "Output (G)"(w384) -> ()
                  }
                }
              }
            }
            n286 = case shown="True" w367 {
              frame False {
                n287 = local read "PID upper\n limit (M)"() -> (w373:dbl)
                n288 = local write "Output (M)"(w373) -> ()
              }
              frame True {
                n289 = local read "PID (M)"() -> (w375:dbl)
                n290 = Less Or Equal?(x=w375, y="PID lower\n limit (M)") -> (x <= y?=w374:bool)
                n291 = case shown="False" w374 {
                  frame False {
                    n292 = local read "PID (M)"() -> (w377:dbl)
                    n293 = local write "Output (M)"(w377) -> ()
                  }
                  frame True {
                    n294 = local read "PID lower\n limit (M)"() -> (w378:dbl)
                    n295 = local write "Output (M)"(w378) -> ()
                  }
                }
              }
            }
          }
          frame #6 {
            w386 = 2.0
            w385 = sgl 1.0 ("WheelSpeed")
            n296 = local read "Current Battery-Driver\nof Motor (A)"() -> (w411:dbl)
            n297 = local read "Current Battery-Driver\nof Generator (A)"() -> (w407:dbl)
            n298 = local read "Lowpass Motor Voltage"() -> (w400:dbl)
            n299 = local read "Lowpass Battery Voltage"() -> (w392:dbl)
            n300 = local read "Current\nDriver-Motor (A)"() -> (w410:dbl)
            n301 = local read "Current\nDriver-Generator (A)"() -> (w408:dbl)
            n302 = local read "Generator Moment (Nm)"() -> (→"Generator Moment Chart":dbl)
            n303 = local read "Calibrated \nmax current"() -> (w417:dbl)
            n304 = local read "Current\nDriver-Generator (A)"() -> (w397:dbl)
            n305 = local read "Calibrated \nmax voltage"() -> (w401:dbl)
            n306 = local read "Motor Moment (Nm)"() -> (→"Motor Moment Chart":dbl)
            n307 = local read "Output (Gen)"() -> (→"Output (Gen)":dbl)
            n308 = local read "Output (Mot)"() -> (→"Output (Mot)":dbl)
            n309 = local read "Lowpass Motor Voltage"() -> (w399:dbl)
            n310 = local read "Motor\nVoltage (V)"() -> (w402:dbl)
            n311 = local read "Generator\nCurrent (A)"() -> (w418:dbl)
            n312 = shared-variable "NI-myRIO-BOSCH-HCMUT\\myRIO_SVs.lvlib\\Boolean"("Boolean") -> ()  [unwired: 1 in, 1 out]
            n313 = local read "Error OUT (G)"() -> (w414:dbl)
            n314 = local read "Error IN (G)"() -> (w412:dbl)
            n315 = Divide(x=w385, y="Ratio") -> (x/y=w389:sgl)
            "?" <- w389
            n316 = Divide(x=w418, y=w417) -> (x/y=w416:dbl)
            n317 = Divide(x=w397, y=w417) -> (x/y=w415:dbl)
            n318 = Merge Signals(w408, w407) -> (→"Generator Current Chart":dynamicdata)
            n319 = Divide(x=w386, y=w389) -> (x/y=→"Slip" →"?":dbl)
            n320 = Divide(x=w402, y=w401) -> (x/y=w405:dbl)
            n321 = Divide(x=w400, y=w401) -> (x/y=w404:dbl)
            n322 = Merge Signals(w410, w411) -> (→"Motor Current Chart":dynamicdata)
            n323 = Merge Signals(w385, w386, w389) -> (→"Speed Chart":dynamicdata)
            n324 = Merge Signals(w399, w392) -> (→"Voltage Chart":dynamicdata)
            n325 = Merge Signals(w412, w414) -> (→"Error Chart":dynamicdata)
            n326 = Merge Signals(w416, w415) -> (→"Generator PID Chart":dynamicdata)
            n327 = Merge Signals(w405, w404) -> (→"Motor PID Chart":dynamicdata)
            "?" <- w386
          }
          frame #7 {
            n328 = local read "Sum ADC Gen Loadcell"() -> (w429:dbl)
            n329 = local read "Sum ADC Mot Loadcell"() -> (w430:dbl)
            n330 = local read "Generator Moment (Nm)"() -> (w422:dbl)
            n331 = local read "Motor Moment (Nm)"() -> (w426:dbl)
            n332 = local read "Current Battery-Driver\nof Generator (A)"() -> (w435:dbl)
            n333 = local read "Sum Mot Moment"() -> (w424:dbl)
            n334 = local read "Sum Gen Moment"() -> (w421:dbl)
            n335 = local read "Current Battery-Driver\nof Motor (A)"() -> (w441:dbl)
            n336 = local read "Lowpass Battery Voltage"() -> (w443:dbl)
            n337 = local read "Lowpass Motor Voltage"() -> (w447:dbl)
            n338 = local read "Current\nDriver-Generator (A)"() -> (w438:dbl)
            n339 = local read "Current\nDriver-Motor (A)"() -> (w452:dbl)
            n340 = local read "Sum Bat-Dri of Mot"() -> (w440:dbl)
            n341 = local read "Sum Bat-Dri of Gen"() -> (w434:dbl)
            n342 = local read "ADC B/AI1"() -> (w427:dbl)
            n343 = local read "ADC B/AI0"() -> (w428:dbl)
            n344 = local read "Sum Generator"() -> (w437:dbl)
            n345 = local read "Sum Speed"() -> (→"Sum Speed":dbl)
            n346 = local read "Sum Motor"() -> (w451:dbl)
            n347 = local read "Samples"() -> (w449:dbl)
            n348 = local read "Sum Mot Voltage"() -> (w446:dbl)
            n349 = local read "Sum Bat Voltage"() -> (w444:dbl)
            n350 = Add(x=w427, y=w429) -> (x+y=→"Sum ADC Gen Loadcell":dbl)
            n351 = Add(x=w428, y=w430) -> (x+y=→"Sum ADC Mot Loadcell":dbl)
            n352 = Add(x=w426, y=w424) -> (x+y=→"Sum Mot Moment":dbl)
            n353 = Add(x=w422, y=w421) -> (x+y=→"Sum Gen Moment":dbl)
            n354 = Increment(x=w449) -> (x+1=→"Samples":dbl)
            n355 = Add(x=w452, y=w451) -> (x+y=→"Sum Motor":dbl)
            n356 = Add(x=w438, y=w437) -> (x+y=→"Sum Generator":dbl)
            n357 = Add(x=w441, y=w440) -> (x+y=→"Sum Bat-Dri of Mot":dbl)
            n358 = Add(x=w435, y=w434) -> (x+y=→"Sum Bat-Dri of Gen":dbl)
            n359 = Add(x=w447, y=w446) -> (x+y=→"Sum Mot Voltage":dbl)
            n360 = Add(x=w443, y=w444) -> (x+y=→"Sum Bat Voltage":dbl)
          }
          frame #8 {
            n361 = local read "Samples"() -> (w455:dbl)
            n362 = Greater Or Equal?(x=w455, y=1000.0) -> (x >= y?=w453:bool)
            n363 = case shown="True" w453 {
              frame False {
              }
              frame True {
                n364 = local read "Sum Bat-Dri of Mot"() -> (w486:dbl)
                n365 = local read "Sum Generator"() -> (w484:dbl)
                n366 = local read "Sum ADC Mot Loadcell"() -> (w466:dbl)
                n367 = local read "Sum Bat Voltage"() -> (w480:dbl)
                n368 = local read "Sum Bat-Dri of Gen"() -> (w482:dbl)
                n369 = local read "Sum Mot Voltage"() -> (w478:dbl)
                n370 = local read "Sum Motor"() -> (w488:dbl)
                n371 = local read "Sum Speed"() -> (w476:dbl)
                n372 = local read "Sum ADC Gen Loadcell"() -> (w464:dbl)
                n373 = local read "Samples"() -> (w475:dbl)
                n374 = local read "Samples"() -> (w487:dbl)
                n375 = local read "Samples"() -> (w479:dbl)
                n376 = local read "Samples"() -> (w467:dbl)
                n377 = local read "Samples"() -> (w465:dbl)
                n378 = local read "Sum Mot Moment"() -> (w461:dbl)
                n379 = local read "Sum Gen Moment"() -> (w459:dbl)
                n380 = local read "Samples"() -> (w477:dbl)
                n381 = local read "Samples"() -> (w483:dbl)
                n382 = local read "Samples"() -> (w485:dbl)
                n383 = local read "Samples"() -> (w481:dbl)
                n384 = Divide(x=w488, y=w487) -> (x/y=→"AVG Current\nDriver-Motor (A)":dbl)
                n385 = local read "Samples"() -> (w460:dbl)
                n386 = local read "Samples"() -> (w458:dbl)
                n387 = Divide(x=w476, y=w475) -> (x/y=→"AVG Speed (RPM)":dbl)
                n388 = Divide(x=w478, y=w477) -> (x/y=→"AVG Voltage Motor (V)":dbl)
                n389 = Divide(x=w486, y=w485) -> (x/y=→"AVG Current Battery-Driver \nof Motor (A)":dbl)
                n390 = Divide(x=w484, y=w483) -> (x/y=→"AVG Current \nDriver-Generator (A)":dbl)
                n391 = Divide(x=w480, y=w479) -> (x/y=→"AVG Voltage Battery (V)":dbl)
                n392 = Divide(x=w482, y=w481) -> (x/y=→"AVG Current Battery-Driver \nof Generator (A)":dbl)
                n393 = Divide(x=w466, y=w467) -> (x/y=→"AVG ADC Mot Loadcell (V)":dbl)
                n394 = Divide(x=w464, y=w465) -> (x/y=→"AVG ADC Gen Loadcell (V)":dbl)
                n395 = Divide(x=w461, y=w460) -> (x/y=→"AVG Motor Moment (Nm)":dbl)
                n396 = Divide(x=w459, y=w458) -> (x/y=→"AVG Generator Moment (Nm)":dbl)
              }
            }
          }
          frame #9 {
            n397 = case shown="True" w489 {
              frame False {
              }
              frame True {
                w492 = 0.0 ("Samples")
                n398 = local read "Generator Moment (Nm)"() -> (w490:dbl)
                n399 = local read "Motor Moment (Nm)"() -> (w491:dbl)
                n400 = local write "Max Gen Moment"(w490) -> ()
                n401 = local write "Max Motor Moment"(w491) -> ()
                n402 = local write "Min Motor Moment"(w491) -> ()
                n403 = local write "Min Gen Moment"(w490) -> ()
                n404 = local write "Sum Bat-Dri of Mot"(w492) -> ()
                n405 = local write "Sum Bat-Dri of Gen"(w492) -> ()
                n406 = local write "Sum Mot Voltage"(w492) -> ()
                n407 = local write "Sum Bat Voltage"(w492) -> ()
                n408 = local write "Sum ADC Mot Loadcell"(w492) -> ()
                n409 = local write "Sum ADC Gen Loadcell"(w492) -> ()
                n410 = local write "Sum Mot Moment"(w492) -> ()
                n411 = local write "Sum Gen Moment"(w492) -> ()
                n412 = local write "Sum Generator"(w492) -> ()
                n413 = local write "Samples"(w492) -> ()
                n414 = local write "Sum Speed"(w492) -> ()
                n415 = local write "Sum Motor"(w492) -> ()
              }
            }
          }
        }
        n416 = call "Tick Count"() -> ("Tick Count(uSec)"=w20:u32)
        n417 = feedback #13() -> (w19:u32)  [unwired: 1 in]
        n418 = feedback-in #13(w20) -> ()
        n419 = Subtract(x=w20, y=w19) -> (x-y=→"Executing Duration":u32)
      }
    }
  }
  n420 = node-c288() -> (w5:T2)  [unwired: 4 in]
  n421 = timed-loop {
    timing: w5 -> [_]
    timing-out: [_] -> w4
    tunnel: w1 -> [w505]
    tunnel: [w494] -> w3
    stop <- FALSE stop-if-true
    n422 = node-c288() -> ()  [unwired: 1 in, 1 out]
    n423 = case shown="True" "PID Generator" {
      tunnel: [w521 w526] -> w493
      frame False {
        n424 = local read "Calibrated \nmax current"() -> (w524:dbl)
        n425 = local read "Generator\nCurrent (A)"() -> (w525:dbl)
        n426 = Divide(x=w525, y=w524) -> (x/y=w523:dbl)
        n427 = Multiply(x=w523, y=100.0) -> (x*y=w521:dbl)
      }
      frame True {
        n428 = local read "Output (G)"() -> (w528:dbl)
        n429 = Multiply(x=w528, y=100.0) -> (x*y=w526:dbl)
      }
    }
    n430 = case shown="False" "PID Motor" {
      tunnel: [w513 w520] -> w501
      frame False {
        n431 = local read "Calibrated \nmax voltage"() -> (w516:dbl)
        n432 = local read "Motor\nVoltage (V)"() -> (w517:dbl)
        n433 = Divide(x=w517, y=w516) -> (x/y=w515:dbl)
        n434 = Multiply(x=w515, y=100.0) -> (x*y=w513:dbl)
      }
      frame True {
        n435 = local read "Output (M)"() -> (w519:dbl)
        n436 = Multiply(x=w519, y=100.0) -> (x*y=w520:dbl)
      }
    }
    n437 = Multiply(x=w493, y=5.0) -> (x*y=w507:dbl)
    n438 = Add(x=w507, y=1500.0) -> (x+y=w510:dbl)
    n439 = To Long Integer(number=w510) -> (32bit integer=w512:i32)
    "32bit integer generator" <- w512
    n440 = Build Array(w512) -> (w511:i32[])
    n441 = xnode "Invoke Method"("FPGA VI Reference In"=w505, "Data"=w511) -> ("FPGA VI Reference Out"=w495:refnum<k20>)  [unwired: 2 in, 2 out]
    n442 = Multiply(x=w501, y=5.0) -> (x*y=w500:dbl)
    n443 = Add(x=w500, y=1500.0) -> (x+y=w497:dbl)
    n444 = To Long Integer(number=w497) -> (32bit integer=w502:i32)
    "32bit integer motor" <- w502
    n445 = Build Array(w502) -> (w503:i32[])
    n446 = xnode "Invoke Method"("FPGA VI Reference In"=w495, "Data"=w503) -> ("FPGA VI Reference Out"=w494:refnum<k20>)  [unwired: 2 in, 2 out]
    n447 = node-c288() -> ()  [unwired: 1 in, 1 out]
  }
  n448 = xnode "Close FPGA VI Reference"("FPGA VI Reference In"=w2) -> ()  [unwired: 1 in, 1 out]
  n449 = node-c288(w4) -> ()  [unwired: 1 out]
  n450 = xnode "Close FPGA VI Reference"("FPGA VI Reference In"=w3) -> ()  [unwired: 1 in, 1 out]
